vi "GDSLvIcon_ReplaceIconColor.vi"(1 "IconIn":u8[][](array[numeric]) format="%x", 2 "OldColor":u32(colorbox), 3 "NewColor":u32(colorbox), 5 "error in (no error)":errorcluster) -> (15 "IconOut":u8[][](array[numeric]) format="%x", 19 "error out":errorcluster)   [LabVIEW 2014]
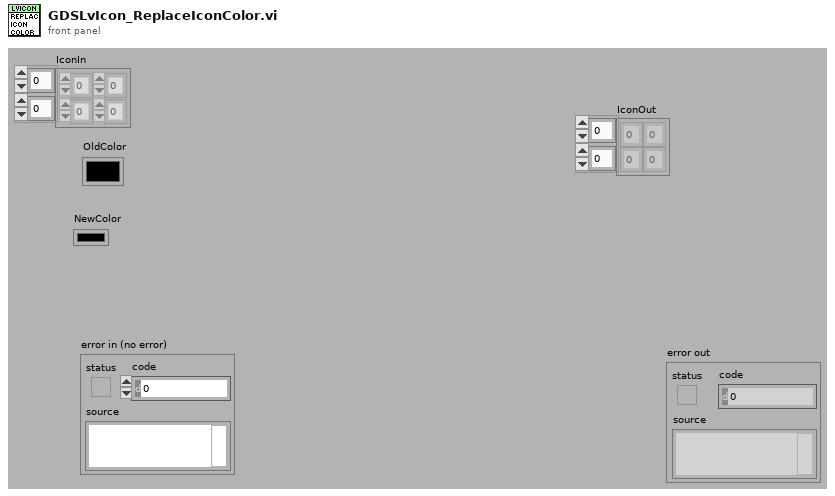
[diagram p1: front panel]
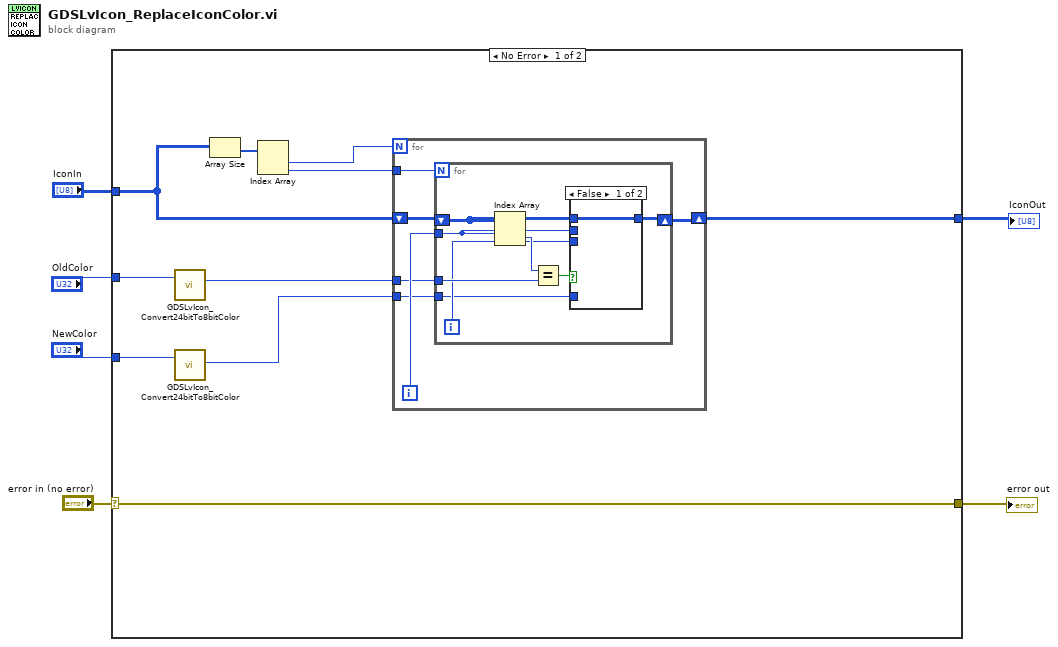
[diagram p0: block diagram]
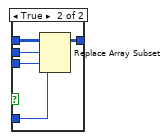
[diagram p2: hidden frame]
diagram:
  n1 = case shown="No Error" "error in (no error)" {
    selector: "error in (no error)" -> [w16 w38]
    tunnel: [w16 w38] -> w5
    tunnel: "OldColor" -> [w15 _]
    tunnel: "NewColor" -> [w14 _]
    tunnel: "IconIn" -> [w10 w37]
    tunnel: [w7 w37] -> w1
    frame No Error {
      n2 = call <resource>:"GDSLvIcon_Convert24bitTo8bitColor.vi"("Color 24bit In"=w15) -> ("Color out(256)"=w9:u8)  [unwired: 15 in, 3 out]
      n3 = call <resource>:"GDSLvIcon_Convert24bitTo8bitColor.vi"("Color 24bit In"=w14) -> ("Color out(256)"=w8:u8)  [unwired: 15 in, 3 out]
      n4 = Array Size(array=w10) -> (size(s)=w13:i32[])
      n5 = Index Array(array=w13) -> (element #1=w12:i32, element #2=w11:i32)  [unwired: 2 in]
      n6 = for {
        N: w12 -> [_]
        shift-right: [w20] -> w7
        shift-left: w10 -> [w22]
        tunnel: w11 -> [w21]
        tunnel: w9 -> [w18]
        tunnel: w8 -> [w17]
        i -> [w19]
        n7 = for {
          N: w21 -> [_]
          shift-right: [w23] -> w20
          shift-left: w22 -> [w27]
          tunnel: w19 -> [w26]
          tunnel: w18 -> [w29]
          tunnel: w17 -> [w24]
          i -> [w25]
          n8 = Index Array(array=w27, index (row)=w26, index (col)=w25) -> (element=w30:u8)
          n9 = Equal?(x=w30, y=w29) -> (x = y?=w28:bool)
          n10 = case shown="False" w28 {
            tunnel: w27 -> [w31 w36]
            tunnel: w26 -> [_ w35]
            tunnel: w25 -> [_ w34]
            tunnel: w24 -> [_ w33]
            tunnel: [w31 w32] -> w23
            frame False {
            }
            frame True {
              n11 = Replace Array Subset(array=w36, new element=w33, index (row)=w35, index (col)=w34) -> (w32:u8[][])
            }
          }
        }
      }
    }
    frame Error {
    }
  }
  "error out" <- w5
  "IconOut" <- w1
